vi "Lab08_Configure_IMAQ.vi"(4 "error in":errorcluster, 5 "Frames":i32, 6 "VideoMode":u32=10, 7 "Session In":T1) -> (0 "error out":errorcluster, 2 "Images Out":T2[](array[typedef]), 3 "Session Out":T1)   [LabVIEW 2021]
doc: "Configures the camera and allocates frame buffers for DAQSP Lab05."
uses:
  <vilib>/userDefined/High Color/IMAQdx.ctl
  <vilib>/vision/Image Controls.llb/IMAQ Image.ctl
  <vilib>/vision/driver/IMAQdx.llb/IMAQdx Acquisition Mode.ctl
  <vilib>/vision/driver/NI_Vision_Acquisition_Software.lvlib
  <resource>/objmgr/imaqdx.rc
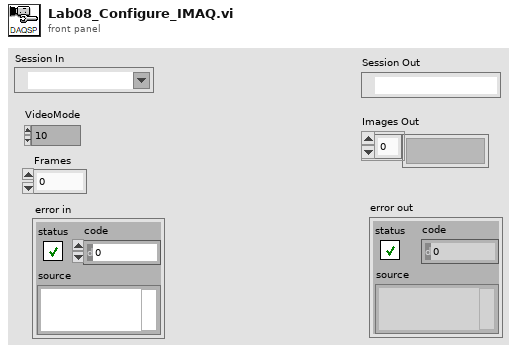
[diagram p1: front panel]
types:
  T1 = typedef "IMAQdx.ctl" = refnum<k21>
  T2 = typedef "IMAQ Image.ctl" = refnum<image>
  T3 = typedef "NI_Vision_Acquisition_Software.lvlib/IMAQdx Acquisition Mode.ctl" = enum32{"One Shot", "Continuous"}
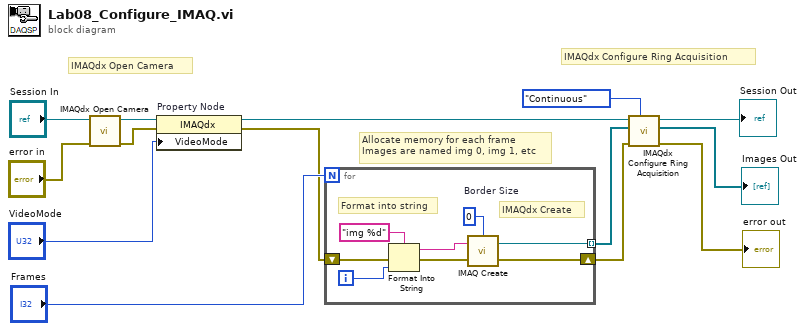
[diagram p0: block diagram]
diagram:
  # "IMAQdx Open Camera"
  # "IMAQdx Configure Ring Acquisition"
  # "Allocate memory for each frame\nImages are named img 0, img 1, etc"
  n1 = call <vilib>:"IMAQdx Open Camera.vi"("error in"="error in", "Session In"="Session In") -> ("error out"=w14:errorcluster, "Session Out"=w13:T1)  [unwired: 1 in, 7 out]
  n2 = property on="Property Node" class="IMAQdx"(reference=w13, error in=w14, "VideoMode"="VideoMode") -> (reference out=w7:T1, error out=w10:errorcluster)
  n3 = for {
    N: "Frames" -> [_]
    tunnel: [w22] -> w8 mode=indexing
    shift-right: [w21] -> w9
    shift-left: w10 -> [w16]
    i -> [w20]
    w17 = 0  # Border Size
    # "IMAQdx Create"
    # "Format into string"
    n4 = Format Into String(format string="img %d" ("Image Name"), error in=w16, w20) -> (resulting string=w19:string, error out=w15:errorcluster)  [unwired: 1 in]
    n5 = call "IMAQ Create"("Border Size"=w17, "Image Name"=w19, "error in (no error)"=w15) -> ("New Image"=w22:T2, "error out"=w21:errorcluster)  [unwired: 1 in, 1 out]
  }
  n6 = call <vilib>:"IMAQdx Configure Ring Acquisition.vi"("Mode"=IMAQdx_Acquisition_Mode."Continuous", "error in"=w9, "Images"=w8, "Session In"=w7) -> ("error out"=→"error out":errorcluster, "Images Out"=→"Images Out":T2[], "Session Out"=→"Session Out":T1)  [unwired: 5 in]
